vi "Activity Log Gen Message Log.vi"(8 "error in (no error)":errorcluster, 10 "Messages":string[](array[string]), 11 "Timestamps":timestamp[](array[timestamp])) -> (0 "error out":errorcluster, 3 "Message Log":string)   [LabVIEW 2021]
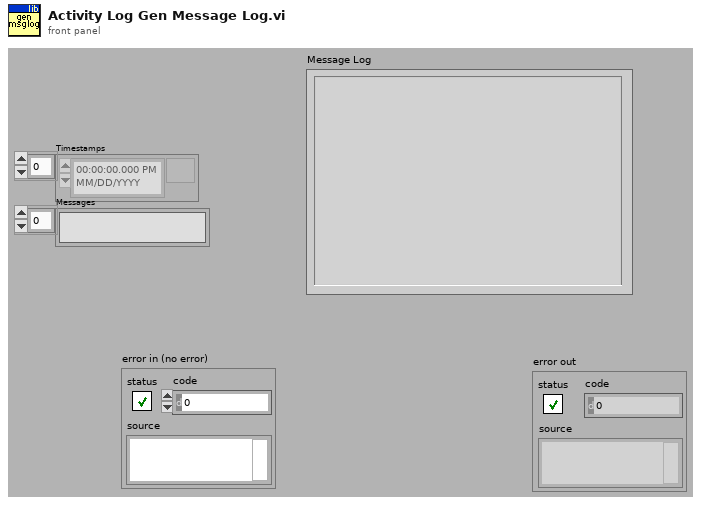
[diagram p1: front panel]
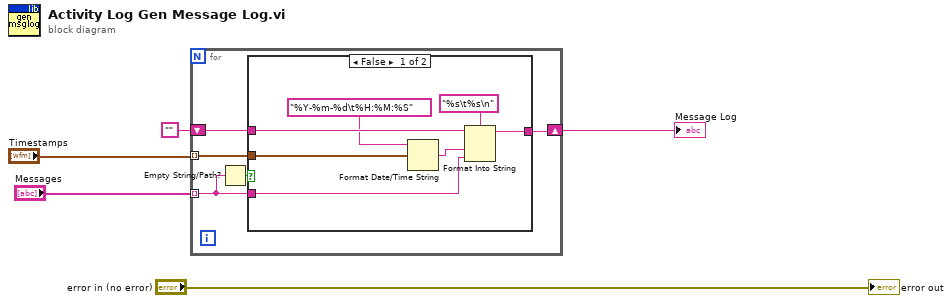
[diagram p0: block diagram]
diagram:
  n1 = for {
    tunnel: "Timestamps" -> [w8] mode=indexing
    tunnel: "Messages" -> [w6] mode=indexing
    shift-right: [w9] -> w3
    shift-left: "" -> [w10]
    n2 = Empty String/Path?(string/path=w6) -> (empty?=w7:bool)
    n3 = case shown="False" w7 {
      tunnel: w10 -> [w16 w18]
      tunnel: w6 -> [w15 _]
      tunnel: [w14 w18] -> w9
      tunnel: w8 -> [w13 _]
      frame False {
        n4 = Format Date/Time String(time format string (%c)="%Y-%m-%d\t%H:%M:%S", seconds (now)=w13) -> (date/time string=w11:string)  [unwired: 1 in]
        n5 = Format Into String(format string="%s\t%s\n", initial string=w16, w11, w15) -> (resulting string=w14:string)  [unwired: 1 in, 1 out]
      }
      frame True {
      }
    }
  }
  "Message Log" <- w3
  "error out" <- "error in (no error)"
